vi "~custom error list.vi"   [LabVIEW 2017]
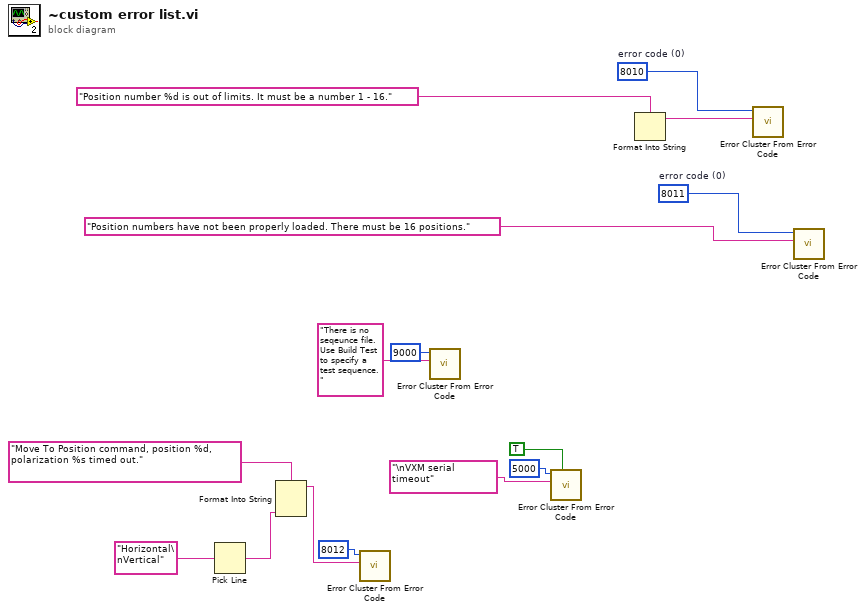
[diagram p0: block diagram]
diagram:
  w10 = 8010  # error code (0)
  w14 = 8011  # error code (0)
  n1 = Pick Line(multi-line string="Horizontal\nVertical" ("format string")) -> (line index=w5:i32, output string=w3:string)  [unwired: 1 in]
  n2 = Format Into String(format string="Move To Position command, position %d, polarization %s timed out.", w3) -> (resulting string=w2:string, w4:i32)  [unwired: 2 in, 1 out]
  n3 = call <vilib>:"Error Cluster From Error Code.vi"("error message (\"\")"=w2, "error code (0)"=8012) -> ("error in (no error)"=w1:errorcluster)  [unwired: 6 in, 1 out]
  n4 = call <vilib>:"Error Cluster From Error Code.vi"("error message (\"\")"="There is no seqeunce file. Use Build Test to specify a test sequence." ("error message (\"\")"), "error code (0)"=9000) -> ("error in (no error)"=w21:errorcluster)  [unwired: 6 in, 1 out]
  n5 = call <vilib>:"Error Cluster From Error Code.vi"("show call chain? (False)"=TRUE, "error message (\"\")"="\nVXM serial timeout" ("ErrorDescription"), "error code (0)"=5000 ("ErrorCode")) -> ("error in (no error)"=w15:errorcluster)  [unwired: 5 in, 1 out]
  n6 = Format Into String(format string="Position number %d is out of limits. It must be a number 1 - 16.") -> (resulting string=w12:string, w11:i32)  [unwired: 2 in, 1 out]
  n7 = call <vilib>:"Error Cluster From Error Code.vi"("error message (\"\")"=w12, "error code (0)"=w10) -> ()  [unwired: 7 in, 1 out]
  n8 = call <vilib>:"Error Cluster From Error Code.vi"("error message (\"\")"="Position numbers have not been properly loaded. There must be 16 positions." ("format string"), "error code (0)"=w14) -> ()  [unwired: 7 in, 1 out]
